vi "Array Manipulation.vi"() -> ()   [LabVIEW 2014]
doc: "本VI演示了不同的处理数据的数组函数。也有范例演示了如何使用LabVIEW内置的多态功能便捷地修改数组中的数据。\n\n检查不同分支，读取程序框图中的说明以了解更多信息。"
uses:
  <vilib>/measure/NI_MABase.lvlib
panel:
  in  "停止按钮":bool
  in  "选项卡控件":T1(tab)
  out "连接的数据数组":dbl[](array[numeric])
  out "连接的数据":dbl[](graph)
  in  "减？":bool
  out "加/减数据数组":dbl[](array[numeric])
  out "加/减数据":dbl[](graph)
  in  "选择通道":u16(ring) items=["通道0", "通道1"]
  out "数据数组的单通道":dbl[](array[numeric])
  out "数据的单通道":dbl[](graph)
  out "数组大小":i32
  in  "偏移量":dbl(slide)=-8.326672684688674e-17 scale=-5.0..5.0
  out "波形数据":waveform(dbl)[](graph)
  out "数据通道数组":dbl[][](array[numeric])
  in  "通道1偏移量":dbl(slide)=-8.326672684688674e-17 scale=-5.0..5.0
  out "全部数据通道":dbl[][](graph)
  out "数组大小":i32[](array[numeric])
  out "子集数据数组":dbl[][](array[numeric])
  in  "开始值":i32(slide)=10 scale=0.0..1000.0
  out "子集数据":dbl[][](graph)
  in  "长度":i32(slide)=1000 scale=0.0..1000.0
  # "行"
  # "列"
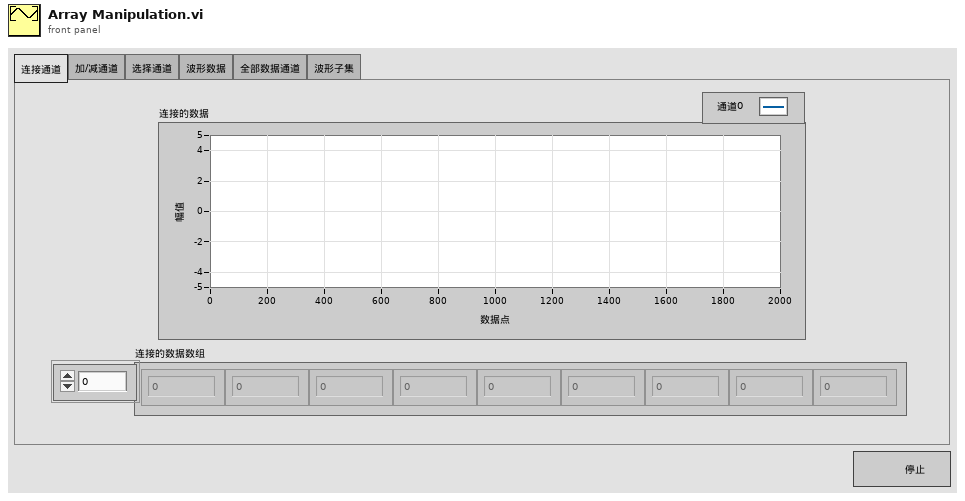
[diagram p1: front panel]
types:
  T1 = enum32{"连接通道", "加/减通道", "选择通道", "波形数据", "全部数据通道", "波形子集"}
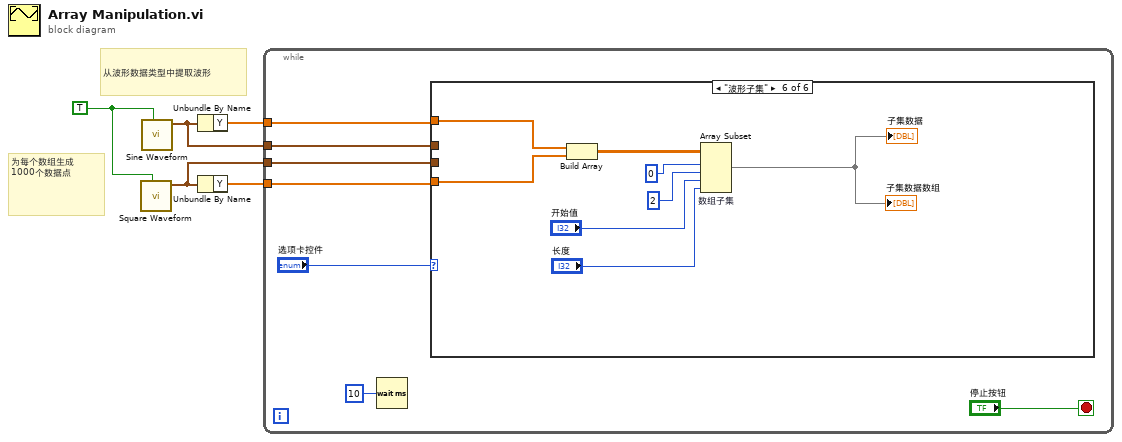
[diagram p0: block diagram]
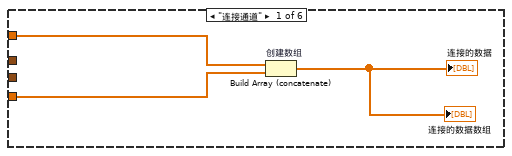
[diagram p2: hidden frame]
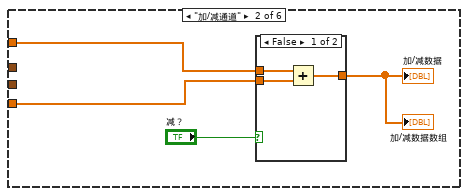
[diagram p3: hidden frame]
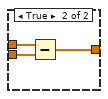
[diagram p4: hidden frame]
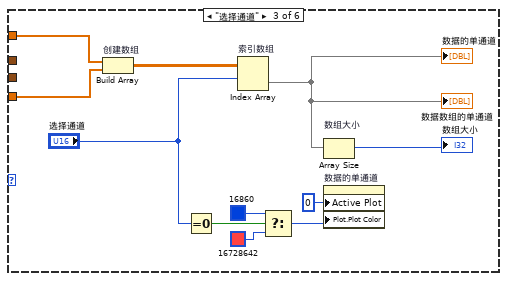
[diagram p5: hidden frame]
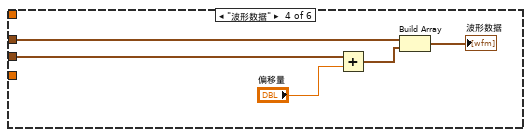
[diagram p6: hidden frame]
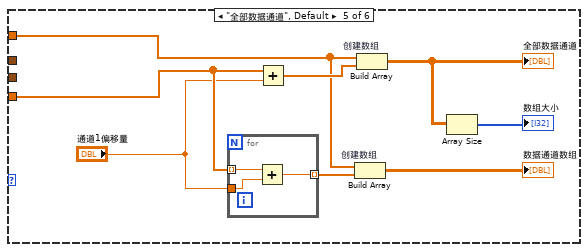
[diagram p7: hidden frame]
diagram:
  w5 = TRUE
  # "从波形数据类型中提取波形"
  # "为每个数组生成\n1000个数据点"
  n1 = call <vilib>:"Square Waveform.vi"("reset signal"=w5) -> ("signal out"=w1:waveform(dbl))  [unwired: 9 in, 1 out]
  n2 = call <vilib>:"Sine Waveform.vi"("reset signal"=w5) -> ("signal out"=w2:waveform(dbl))  [unwired: 9 in, 1 out]
  n3 = Unbundle By Name ("Get Waveform Components")(w2) -> ("Y"=w4:dbl[])
  n4 = Unbundle By Name ("Get Waveform Components")(w1) -> ("Y"=w3:dbl[])
  n5 = while {
    tunnel: w4 -> [w10]
    tunnel: w3 -> [w9]
    tunnel: w2 -> [w8]
    tunnel: w1 -> [w7]
    stop <- "停止按钮" stop-if-true
    n6 = Wait (ms)(milliseconds to wait=u32 10 ("等待时间（毫秒）")) -> ()  [unwired: 1 out]
    n7 = case shown="\"波形子集\"" "选项卡控件" {
      tunnel: w10 -> [w14 w19 w36 _ w45 w60]
      tunnel: w9 -> [w15 w18 w35 _ w48 w59]
      tunnel: w8 -> [_ _ _ w41 _ _]
      tunnel: w7 -> [_ _ _ w37 _ _]
      frame "连接通道" {
        n8 = Build Array (concatenate) "创建数组"(w14, w15) -> (→"连接的数据" →"连接的数据数组":dbl[])
      }
      frame "加/减通道" {
        n9 = case shown="False" "减？" {
          tunnel: w19 -> [w22 w25]
          tunnel: w18 -> [w21 w24]
          tunnel: [w20 w23] -> w16
          frame False {
            n10 = Add(x=w22, y=w21) -> (x+y=w20:dbl[])
          }
          frame True {
            n11 = Subtract(x=w25, y=w24) -> (x-y=w23:dbl[])
          }
        }
        "加/减数据" <- w16
        "加/减数据数组" <- w16
      }
      frame "选择通道" {
        n12 = Build Array "创建数组"(w36, w35) -> (w34:dbl[][])
        n13 = Equal To 0?(x="选择通道") -> (x = 0?=w27:bool)
        n14 = Index Array "索引数组"(array=w34, index (row)="选择通道") -> (element=w33:dbl[])  [unwired: 1 in]
        "数据的单通道" <- w33
        "数据数组的单通道" <- w33
        n15 = Select(t=u32 16860, s=w27, f=u32 16728642) -> (s? t:f=w30:u32)
        n16 = Array Size "数组大小"(array=w33) -> (size(s)=→"数组大小":i32)
        n17 = property on="数据的单通道" class="WFGraph (strict)"("Active Plot"=u32 0 ("活动曲线"), "Plot.Plot Color"=w30) -> ()  [unwired: 2 in, 2 out]
      }
      frame "波形数据" {
        n18 = Add(x=w37, y="偏移量") -> (x+y=w40:waveform(dbl))
        n19 = Build Array(w41, w40) -> (→"波形数据":waveform(dbl)[])
      }
      frame "全部数据通道", Default {
        n20 = for {
          tunnel: w48 -> [w52] mode=indexing
          tunnel: "通道1偏移量" -> [w51]
          tunnel: [w50] -> w46 mode=indexing
          n21 = Add(x=w52, y=w51) -> (x+y=w50:dbl)
        }
        n22 = Add(x=w48, y="通道1偏移量") -> (x+y=w49:dbl[])
        n23 = Build Array "创建数组"(w45, w46) -> (→"数据通道数组":dbl[][])
        n24 = Build Array "创建数组"(w45, w49) -> (w43:dbl[][])
        "全部数据通道" <- w43
        n25 = Array Size(array=w43) -> (size(s)=→"数组大小":i32[])
      }
      frame "波形子集" {
        n26 = Build Array(w60, w59) -> (w58:dbl[][])
        n27 = Array Subset "数组子集"(array=w58, index (row)=0 ("索引"), length (row)=2 ("长度"), index (col)="开始值", length (col)="长度") -> (→"子集数据数组" →"子集数据":dbl[][])
      }
    }
  }
